vi "1.vi"() -> ()   [LabVIEW 2020]
panel:
  out "Waveform Graph 2":dbl[](graph)
  in  "stop":bool
  out "Waveform Chart":dbl(graph)
  in  "dx":dbl
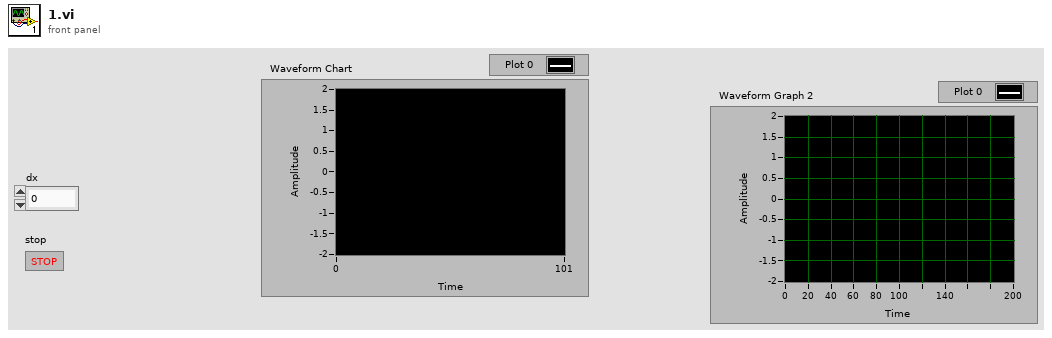
[diagram p1: front panel]
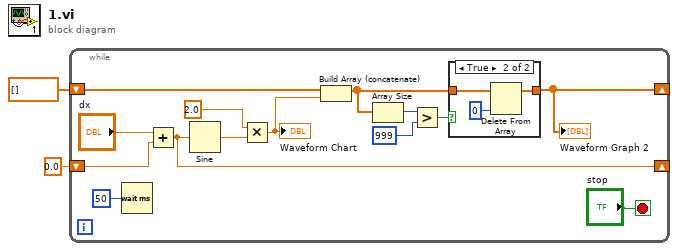
[diagram p0: block diagram]
diagram:
  n1 = while {
    shift-right: [w14] -> _
    shift-left: 0.0 -> [w3]
    shift-right: [w5] -> _
    shift-left: dbl[] [] -> [w10]
    stop <- "stop" stop-if-true
    n2 = Wait (ms)(milliseconds to wait=u32 50 ("millisecond timer value")) -> ()  [unwired: 1 out]
    n3 = Add(x="dx", y=w3) -> (x+y=w14:dbl)
    n4 = Sine(x=w14) -> (sin(x)=w16:dbl)
    n5 = Multiply(x=2.0, y=w16) -> (x*y=w11:dbl)
    "Waveform Chart" <- w11
    n6 = Build Array (concatenate)(w10, w11) -> (w6:dbl[])
    n7 = Array Size(array=w6) -> (size(s)=w9:i32)
    n8 = Greater?(x=w9, y=999) -> (0:w7:bool)
    n9 = case shown="True" w7 {
      tunnel: w6 -> [w17 w20]
      tunnel: [w17 w18] -> w5
      frame False {
      }
      frame True {
        n10 = Delete From Array(array=w20, index=0) -> (array with subset deleted=w18:dbl[])  [unwired: 1 in, 1 out]
      }
    }
    "Waveform Graph 2" <- w5
  }
